vi "Volume Pull Collect.vi"(7 "Notifier Data":T2, 8 "error in (no error)":errorcluster, 10 "Data Cluster":T1, 11 "Notifier in":refnum<notifier>) -> (0 "error out":errorcluster, 1 "Free Air Flow Data":dbl[][](array[numeric]), 2 "STOP Button Pressed":bool, 3 "Timeout":bool, 4 "Stabilzed Pressure":dbl, 5 "Pressure Stabilized":bool)   [LabVIEW 2026, in "Acquisition.lvlib"]
uses:
  Acquisition.lvlib
  controls/NotifierAndDataQueue.ctl
  controls/WaveformChartData.ctl
  Hardware Configuration.ctl
  Settings/Settings.lvlib
panel:
  out "x-y":dbl
  out "x >= y?":bool
  out "% Change":dbl
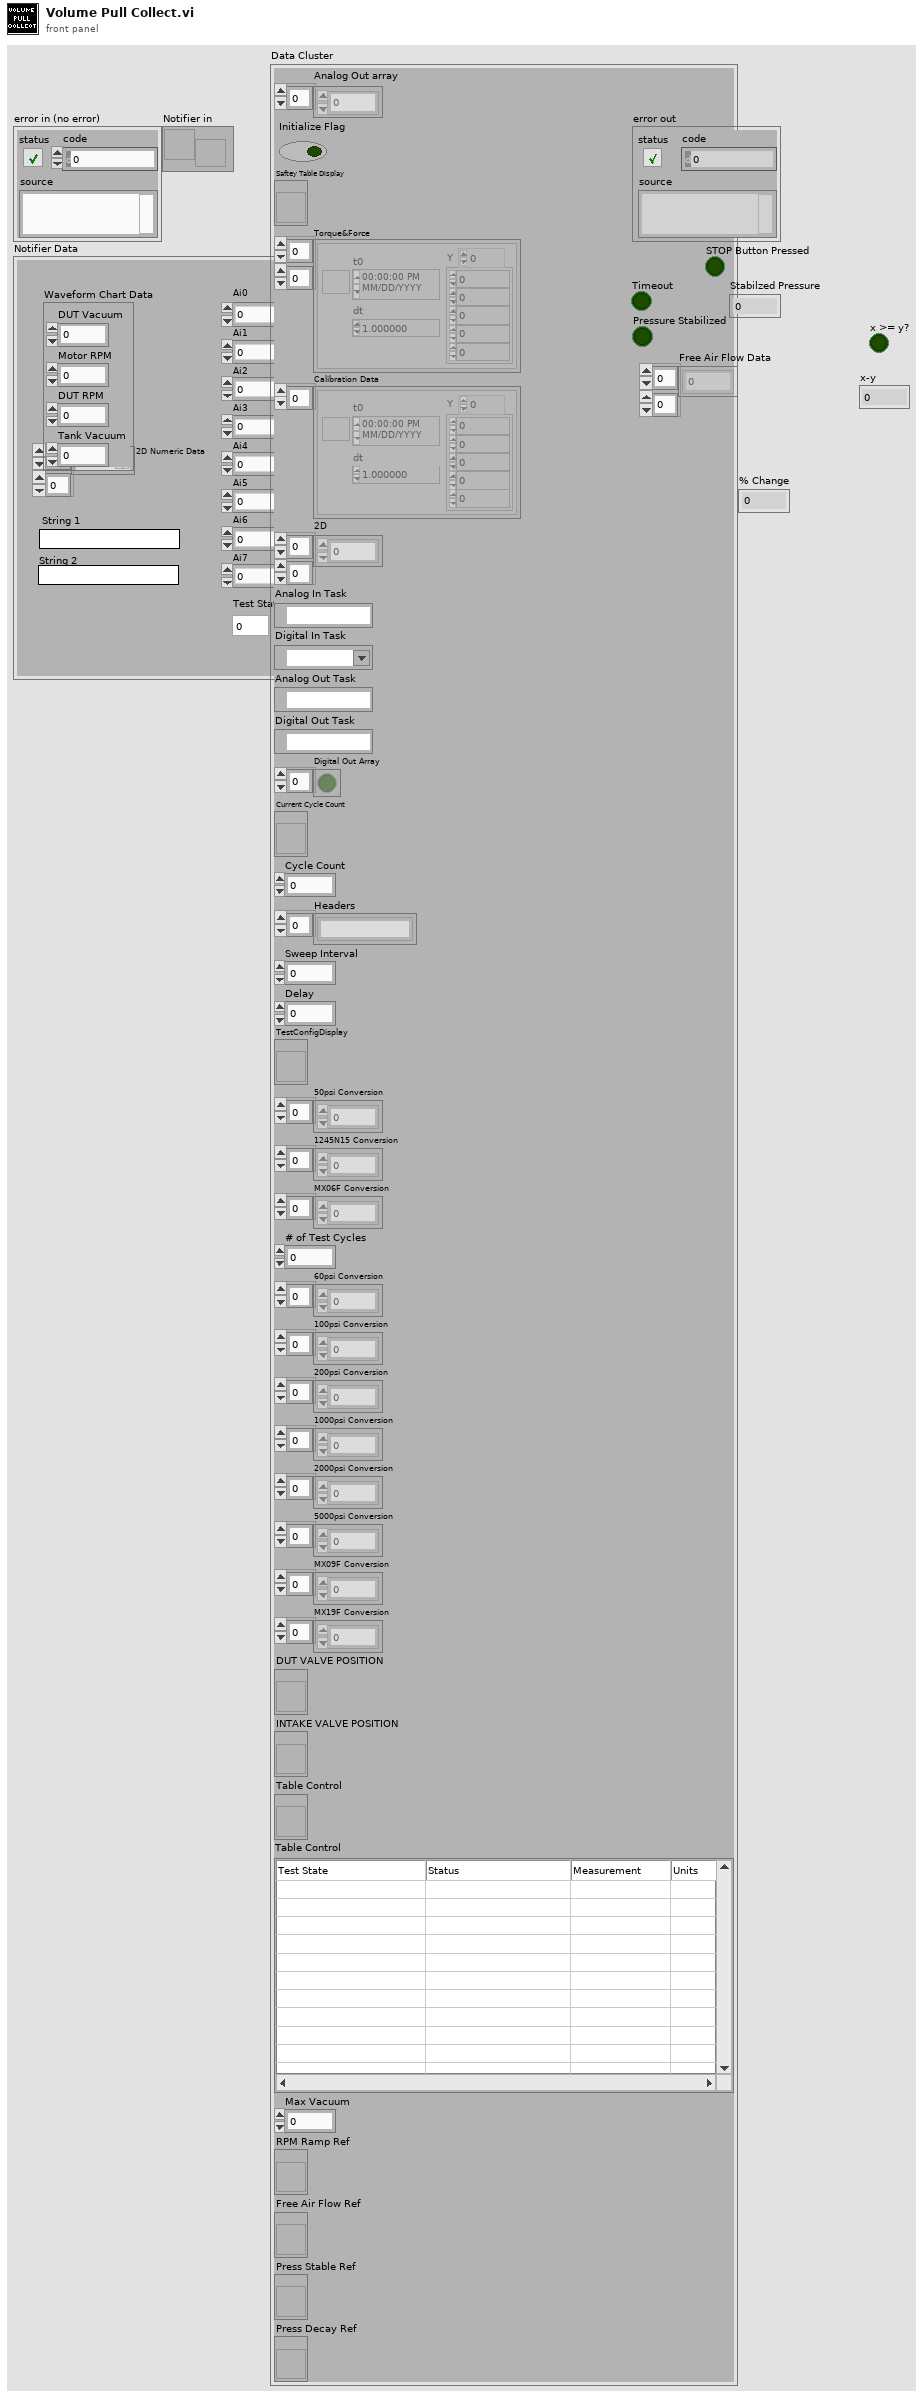
[diagram p1: front panel]
types:
  T1 = typedef "Acquisition.lvlib/Hardware Configuration.ctl" = cluster{"Analog Out array":dbl[], "Initialize Flag":bool, "Saftey Table Display":refnum<vi>, "Torque&Force":waveform(dbl)[][], "Calibration Data":waveform(dbl)[], "2D":dbl[][], "Analog In Task":refnum<k21>, "Digital In Task":refnum<k21>, "Analog Out Task":refnum<k21>, "Digital Out Task":refnum<k21>, "Digital Out Array":bool[], "Current Cycle Count":refnum<vi>, "Cycle Count":u64, "Headers":string[], "Sweep Interval":u64, "Delay":u64, "TestConfigDisplay":refnum<vi>, "50psi Conversion":dbl[], "1245N15 Conversion":dbl[], "MX06F Conversion":dbl[], "# of Test Cycles":u64, "60psi Conversion":dbl[], "100psi Conversion":dbl[], "200psi Conversion":dbl[], "1000psi Conversion":dbl[], "2000psi Conversion":dbl[], "5000psi Conversion":dbl[], "MX09F Conversion":dbl[], "MX19F Conversion":dbl[], "DUT VALVE POSITION":refnum<vi>, "INTAKE VALVE POSITION":refnum<vi>, "Table Control":refnum<vi>, "Table Control":string[][], "Max Vacuum":dbl, "RPM Ramp Ref":refnum<vi>, "Free Air Flow Ref":refnum<vi>, "Press Stable Ref":refnum<vi>, "Press Decay Ref":refnum<vi>}
  T2 = typedef "NotifierAndDataQueue.ctl" = cluster{"Ai0":dbl, "Ai1":dbl, "Ai2":dbl, "Ai3":dbl, "Ai4":dbl, "Ai5":dbl, "Ai6":dbl, "Ai7":dbl, "P0.0":bool, "P0.1":bool, "P0.2":bool, "P0.3":bool, "P0.4":bool, "P0.5":bool, "P0.6":bool, "P0.7":bool, "2D Numeric Data":dbl[][], "String 2":string, "String 1":string, "Waveform Chart Data":T3, "Test State Timer":dbl}
  T3 = typedef "Settings.lvlib/WaveformChartData.ctl" = cluster{"DUT Vacuum":dbl, "Motor RPM":dbl, "DUT RPM":dbl, "Tank Vacuum":dbl}
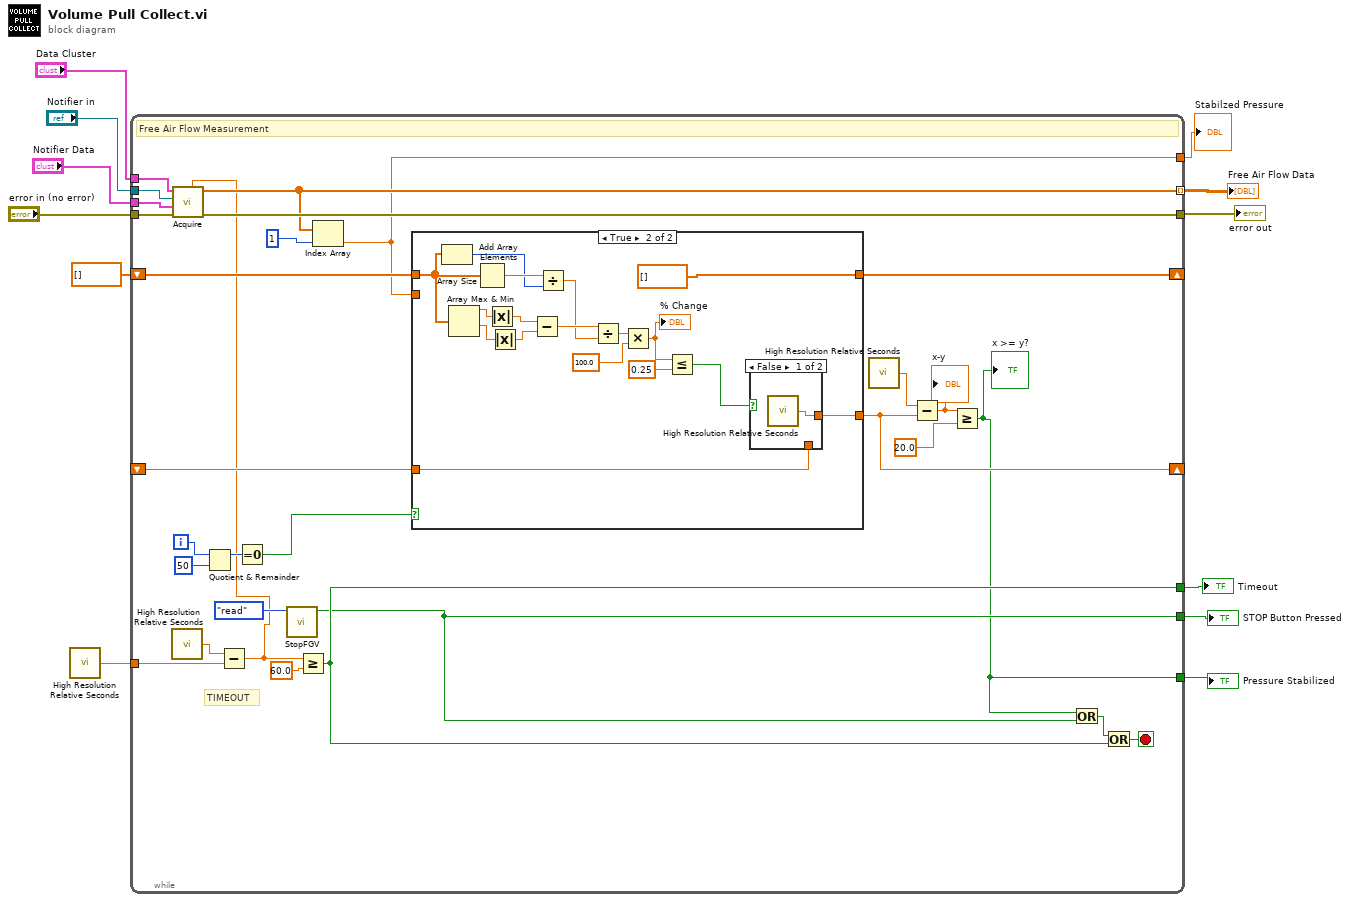
[diagram p0: block diagram]
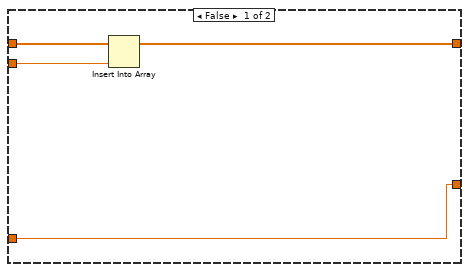
[diagram p2: hidden frame]
diagram:
  n1 = call <vilib>:"High Resolution Relative Seconds.vi"() -> ("relative seconds"=w5:dbl)
  n2 = while {
    tunnel: "Notifier in" -> [w39]
    tunnel: "error in (no error)" -> [w41]
    tunnel: [w40] -> w9
    tunnel: "Notifier Data" -> [w36]
    tunnel: "Data Cluster" -> [w35]
    tunnel: [w21] -> w7
    tunnel: [w32] -> w6
    tunnel: w5 -> [w31]
    tunnel: [w30] -> w4 mode=indexing
    shift-right: [w28] -> _
    shift-left: dbl[] [] -> [w23]
    tunnel: [w15] -> w2
    shift-right: [w17] -> _
    shift-left: _ -> [w18]
    tunnel: [w14] -> w1
    i -> [w27]
    stop <- w37 stop-if-true
    # "TIMEOUT"
    # "Free Air Flow Measurement"
    n3 = call <vilib>:"High Resolution Relative Seconds.vi"() -> ("relative seconds"=w34:dbl)
    n4 = Quotient & Remainder(x=w27, y=50) -> (x-y*floor(x/y)=w25:i32)  [unwired: 1 out]
    n5 = Subtract(x=w34, y=w31) -> (x-y=w13:dbl)
    n6 = call "Acquire.vi"("Test State Timer"=w13, "error in (no error)"=w41, "Notifiier Data"=w36, "notifier out"=w39, "Hardware Resources in"=w35) -> ("error out"=w40:errorcluster, "Averaged Data Array"=w30:dbl[])  [unwired: 4 in, 1 out]
    n7 = Equal To 0?(x=w25) -> (x = 0?=w24:bool)
    n8 = call "StopFGV.vi"("Enum"=enum16{"init", "write", "read"}."read") -> ("STOP Out"=w21:bool)  [unwired: 9 in, 1 out]
    n9 = Greater Or Equal?(x=w13, y=60.0) -> (x >= y?=w32:bool)
    n10 = Index Array(array=w30, index=1) -> (element=w14:dbl)
    n11 = case shown="True" w24 {
      tunnel: w14 -> [w45 _]
      tunnel: [w44 dbl[] []] -> w28
      tunnel: w23 -> [w43 w61]
      tunnel: [w42 w47] -> w17
      tunnel: w18 -> [w42 w46]
      frame False {
        n12 = Insert Into Array(array=w43, new element=w45) -> (w44:dbl[])  [unwired: 1 in]
      }
      frame True {
        n13 = Array Size(array=w61) -> (size(s)=w59:i32)
        n14 = Array Max & Min(array=w61) -> (max value=w58:dbl, min value=w56:dbl)  [unwired: 2 out]
        n15 = Add Array Elements(numeric array=w61) -> (sum=w60:dbl)
        n16 = Absolute Value(x=w58) -> (abs(x)=w57:dbl)
        n17 = Absolute Value(x=w56) -> (abs(x)=w55:dbl)
        n18 = Subtract(x=w57, y=w55) -> (x-y=w54:dbl)
        n19 = Divide(x=w60, y=w59) -> (x/y=w53:dbl)
        n20 = Divide(x=w54, y=w53) -> (x/y=w52:dbl)
        n21 = Multiply(x=w52, y=100.0) -> (x*y=w50:dbl)
        "% Change" <- w50
        n22 = Less Or Equal?(x=w50, y=0.25) -> (x <= y?=w48:bool)
        n23 = case shown="False" w48 {
          tunnel: [w63 w64] -> w47
          tunnel: w46 -> [_ w64]
          frame False {
            n24 = call <vilib>:"High Resolution Relative Seconds.vi"() -> ("relative seconds"=w63:dbl)
          }
          frame True {
          }
        }
      }
    }
    n25 = call <vilib>:"High Resolution Relative Seconds.vi"() -> ("relative seconds"=w20:dbl)
    n26 = Subtract(x=w20, y=w17) -> (x-y=w16:dbl)
    "x-y" <- w16
    n27 = Greater Or Equal?(x=w16, y=20.0) -> (x >= y?=w15:bool)
    "x >= y?" <- w15
    n28 = Or(x=w15, y=w21) -> (x .or. y?=w22:bool)
    n29 = Or(x=w22, y=w32) -> (x .or. y?=w37:bool)
  }
  "error out" <- w9
  "STOP Button Pressed" <- w7
  "Timeout" <- w6
  "Free Air Flow Data" <- w4
  "Pressure Stabilized" <- w2
  "Stabilzed Pressure" <- w1
